vi "fmeasure.vi"(8 "error in (no error)":errorcluster, 11 "Bronkhorst Settings in":T1={"VISA resource name"="", "Simulated?"=FALSE, "Smoothing Steps"=1} {"Smoothing Steps" min=1 step=1}) -> (0 "error out":errorcluster, 1 "Connection Error":bool, 2 "flow":dbl, 3 "Bronkhorst Settings out":T1={"VISA resource name"="", "Simulated?"=FALSE, "Smoothing Steps"=1} {"Smoothing Steps" min=1 step=1}, 4 "*(type *) &x":dbl, 5 "submatch 1":string, 6 "read buffer":string)   [LabVIEW 2021, in "Bronkhorst M14 Flow Meter.lvlib"]
uses:
  Bronkhorst M14 Flow Meter.lvlib
  Settings Cluster.ctl
  <vilib>/regexp/Match Regular Expression.xnode
  <vilib>/ptbypt/NI_PtbyPt.lvlib
panel:
  out "before match":string
  out "whole match":string
  out "x/y":dbl
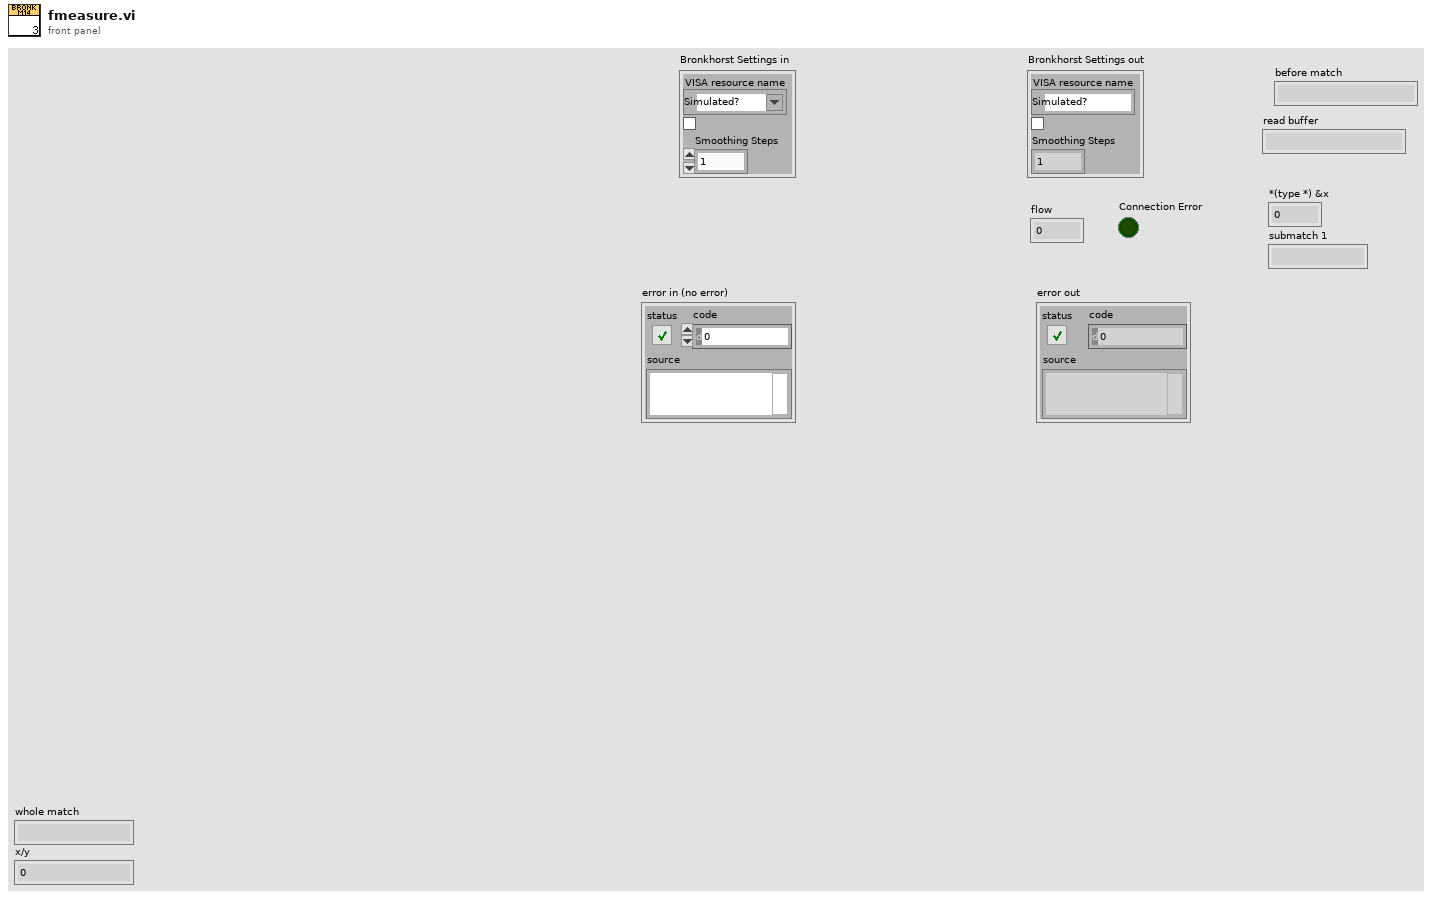
[diagram p1: front panel]
types:
  T1 = typedef "Bronkhorst M14 Flow Meter.lvlib/Settings Cluster.ctl" = cluster{"VISA resource name":refnum<visa-resource-name>, "Simulated?":bool, "Smoothing Steps":i32}
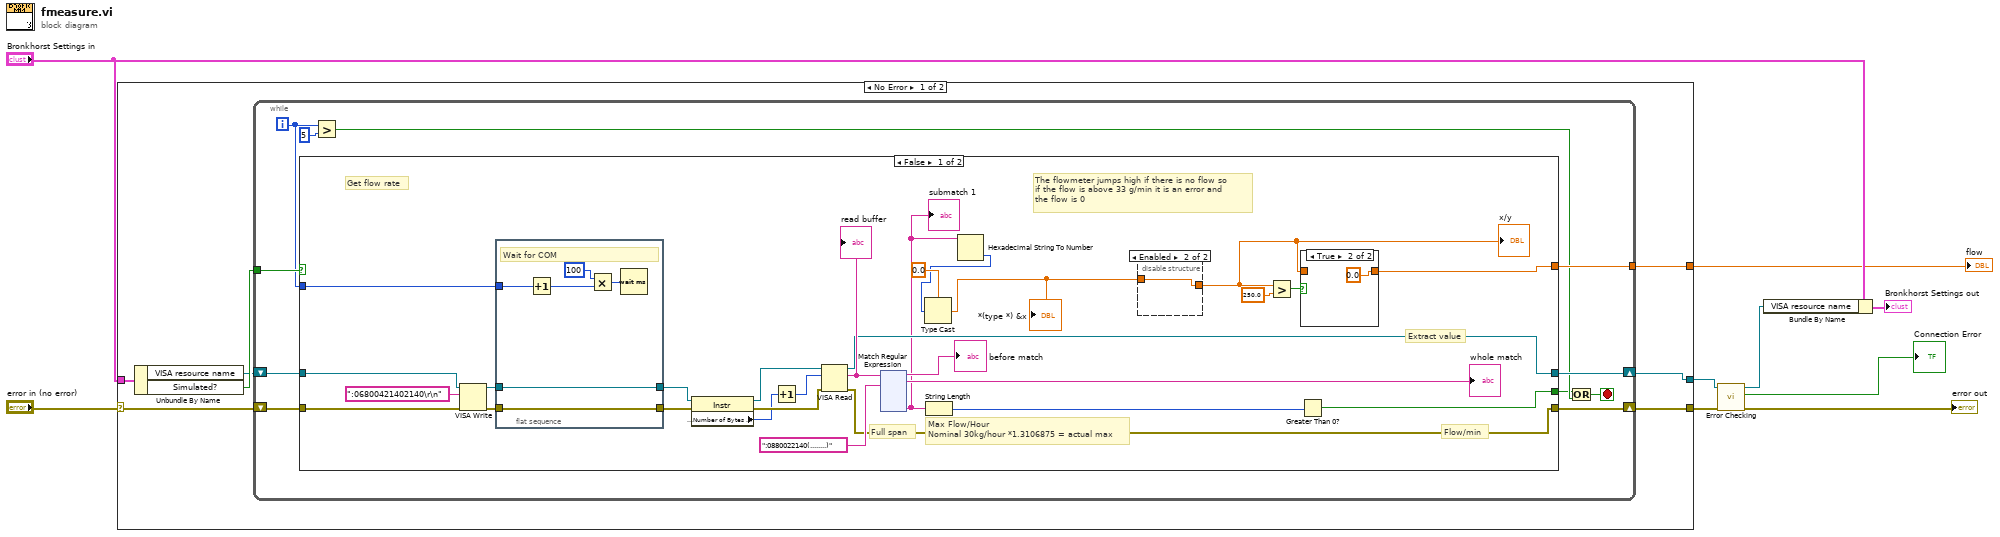
[diagram p0: block diagram]
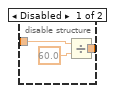
[diagram p2: hidden frame]
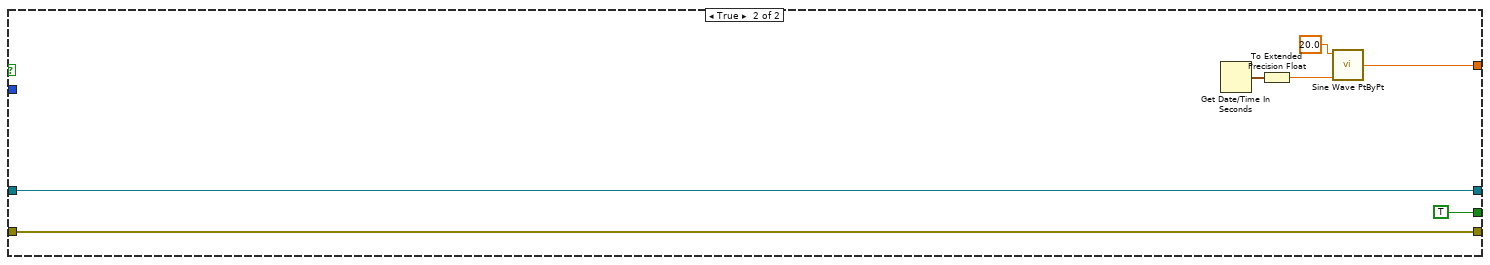
[diagram p4: hidden frame]
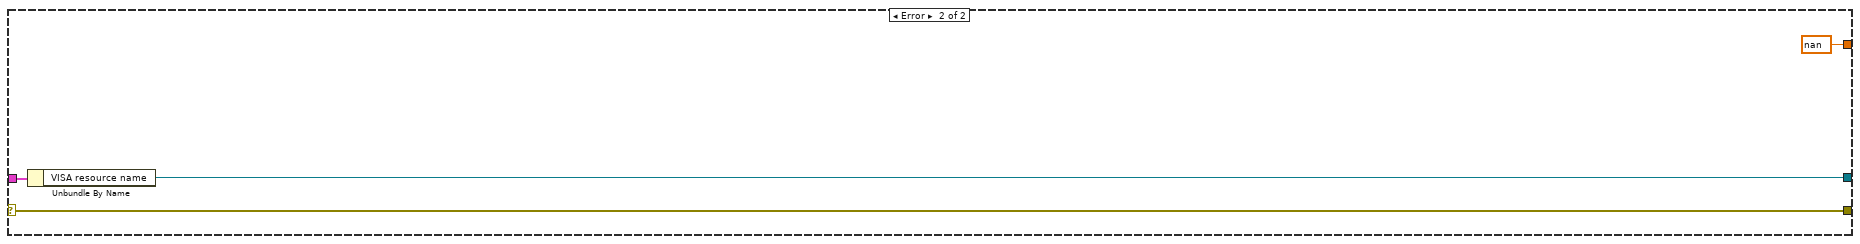
[diagram p5: hidden frame]
diagram:
  n1 = case shown="No Error" "error in (no error)" {
    selector: "error in (no error)" -> [w15 w197]
    tunnel: [w14 w197] -> w7
    tunnel: "Bronkhorst Settings in" -> [w12 w195]
    tunnel: [w13 nan ("sine wave")] -> w4
    tunnel: [w10 w194] -> w9
    frame No Error {
      n2 = Unbundle By Name(w12) -> ("VISA resource name"=w11:refnum<visa-resource-name>, "Simulated?"=w16:bool)
      n3 = while {
        tunnel: w16 -> [w27]
        tunnel: [w24] -> w13
        shift-right: [w25] -> w14
        shift-left: w15 -> [w26]
        shift-right: [w22] -> w10
        shift-left: w11 -> [w23]
        i -> [w18]
        stop <- w17 stop-if-true
        n4 = case shown="False" w27 {
          tunnel: [w36 w193] -> w25
          tunnel: w26 -> [w41 w193]
          tunnel: [w44 w189] -> w24
          tunnel: [w37 w188] -> w22
          tunnel: w23 -> [w42 w188]
          tunnel: [w33 TRUE] -> w19
          tunnel: w18 -> [w35 _]
          frame False {
            # "Flow/min"
            # "Max Flow/Hour\nNominal 30kg/hour *1.3106875 = actual max"
            # "Full span"
            # "Extract value"
            # "Get flow rate"
            # "The flowmeter jumps high if there is no flow so \nif the flow is above 33 g/min it is an error and \nthe flow is 0"
            n5 = VISA Write(VISA resource name=w42, write buffer=":06800421402140\r\n" ("Command"), error in (no error)=w41) -> (VISA resource name out=w52:refnum<visa-resource-name>, error out=w50:errorcluster)  [unwired: 1 out]
            n6 = flat-sequence {
              tunnel: [w186] -> w51
              tunnel: w52 -> [w186]
              tunnel: [w185] -> w49
              tunnel: w50 -> [w185]
              tunnel: w35 -> [w182]
              frame #0 {
                # "Wait for COM"
                n7 = Increment(x=w182) -> (x+1=w181:i32)
                n8 = Multiply(x=u32 100 ("milliseconds to wait"), y=w181) -> (x*y=w183:u32)
                n9 = Wait (ms)(milliseconds to wait=w183) -> ()  [unwired: 1 out]
              }
            }
            n10 = property class="Instr"(reference=w51, error in=w49) -> (reference out=w54:refnum<visa-resource-name>, error out=w53:errorcluster, "Serial Settings:Number of Bytes at Serial Port"=w39:u32)
            n11 = Increment(x=w39) -> (x+1=w38:u32)
            n12 = VISA Read(VISA resource name=w54, byte count=w38, error in (no error)=w53) -> (VISA resource name out=w37:refnum<visa-resource-name>, read buffer=w40:string, error out=w36:errorcluster)  [unwired: 1 out]
            "read buffer" <- w40
            n13 = xnode "Match Regular Expression"("input string"=w40, "regular expression"=":0880022140(........)" ("Regular Expression for Extracting Weight")) -> ("before match"=→"before match":string, "whole match"=→"whole match":string, "submatch 1"=w28:string)  [unwired: 4 in, 3 out]
            "submatch 1" <- w28
            n14 = String Length(string=w28) -> (length=w34:i32)
            n15 = Hexadecimal String To Number(string=w28) -> (number=w29:u32)  [unwired: 2 in, 1 out]
            n16 = Type Cast(type=0.0, x=w29) -> (*(type *) &x=w31:dbl)
            "*(type *) &x" <- w31
            n17 = disable-structure shown="Enabled" {
              disable-tunnel: [w57 w59] -> w45
              disable-tunnel: w31 -> [w56 w59]
              frame Disabled {
                n18 = Divide(x=w56, y=60.0) -> (x/y=w57:dbl)
              }
              frame Enabled {
              }
            }
            "x/y" <- w45
            n19 = Greater?(x=w45, y=250.0) -> (0:w46:bool)
            n20 = Greater Than 0?(x=w34) -> (x > 0?=w33:bool)
            n21 = case shown="True" w46 {
              tunnel: [w60 0.0] -> w44
              tunnel: w45 -> [w60 _]
              frame False {
              }
              frame True {
              }
            }
          }
          frame True {
            n22 = Get Date/Time In Seconds() -> (seconds since 1Jan1904=w192:timestamp)
            n23 = To Extended Precision Float(1:w192) -> (0:w191:ext)
            n24 = call <vilib>:"Sine Wave PtByPt.vi"("time"=w191, "amplitude"=20.0) -> ("sine wave"=w189:dbl)  [unwired: 2 in]
          }
        }
        n25 = Greater?(x=w18, y=5) -> (0:w20:bool)
        n26 = Or(x=w19, y=w20) -> (x .or. y?=w17:bool)
      }
    }
    frame Error {
      n27 = Unbundle By Name(w195) -> ("VISA resource name"=w194:refnum<visa-resource-name>)
    }
  }
  "flow" <- w4
  n28 = call "Error Checking.vi"("error in (no error)"=w7, "VISA resource name"=w9) -> ("error out"=→"error out":errorcluster, "Connection Error"=→"Connection Error":bool, "VISA resource name"=w8:refnum<visa-resource-name>)  [unwired: 7 in]
  n29 = Bundle By Name(cluster="Bronkhorst Settings in", "VISA resource name"=w8) -> (→"Bronkhorst Settings out":T1)
